vi "Init.vi"(8 "error in (no error)":errorcluster, 11 "Camera View in":refnum<class "Camera View.lvclass">) -> (0 "error out":errorcluster, 3 "Camera View out":refnum<class "Camera View.lvclass">)   [LabVIEW 2022 SP3, in "Camera View.lvclass"]
uses:
  Camera View.lvclass
  iView/base view/base view.lvclass
  Camera View.lvclass/Camera View.ctl
  Camera Controller/Camera Controller.lvclass
  Data.ctl
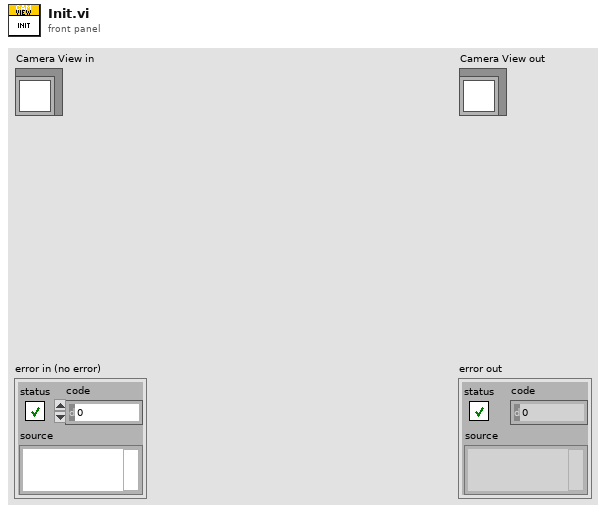
[diagram p1: front panel]
types:
  T1 = typedef "Camera View.lvclass/Data.ctl" = cluster{"Camera Controller.lvclass":refnum<class "Camera Controller.lvclass">}
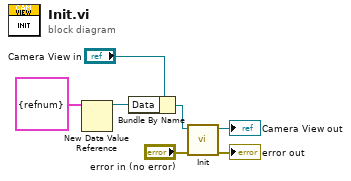
[diagram p0: block diagram]
diagram:
  n1 = New Data Value Reference(data value=T1 {"Camera Controller.lvclass"=refnum} ("Data")) -> (data value reference=w1:refnum<data-value>)  [unwired: 1 in, 1 out]
  n2 = Bundle By Name(cluster="Camera View in", "Data"=w1) -> (w2:refnum<class "Camera View.lvclass">)
  n3 = call-parent "Init.vi"("error in (no error)"="error in (no error)", "base view in"=w2) -> ("error out"=→"error out":errorcluster, "base view out"=→"Camera View out":refnum<class "Camera View.lvclass">)  [unwired: 8 in]
